vi "WhiteScreenTest_Startup.vi"() -> (0 "ErrorOut":errorcluster)   [LabVIEW 2018] (continued)
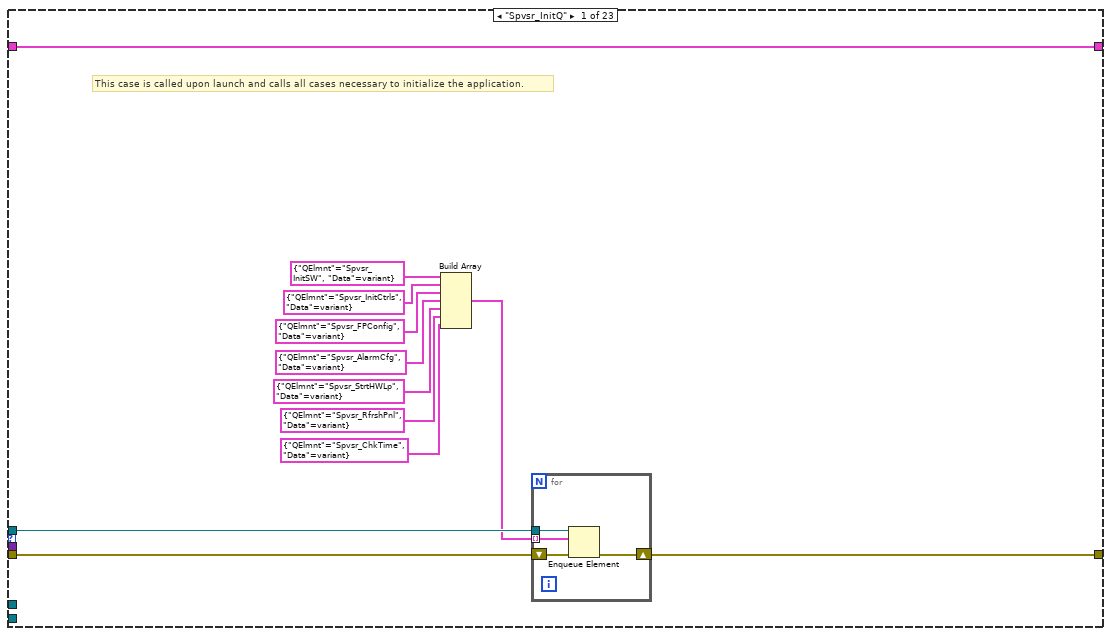
[diagram p6: hidden frame]
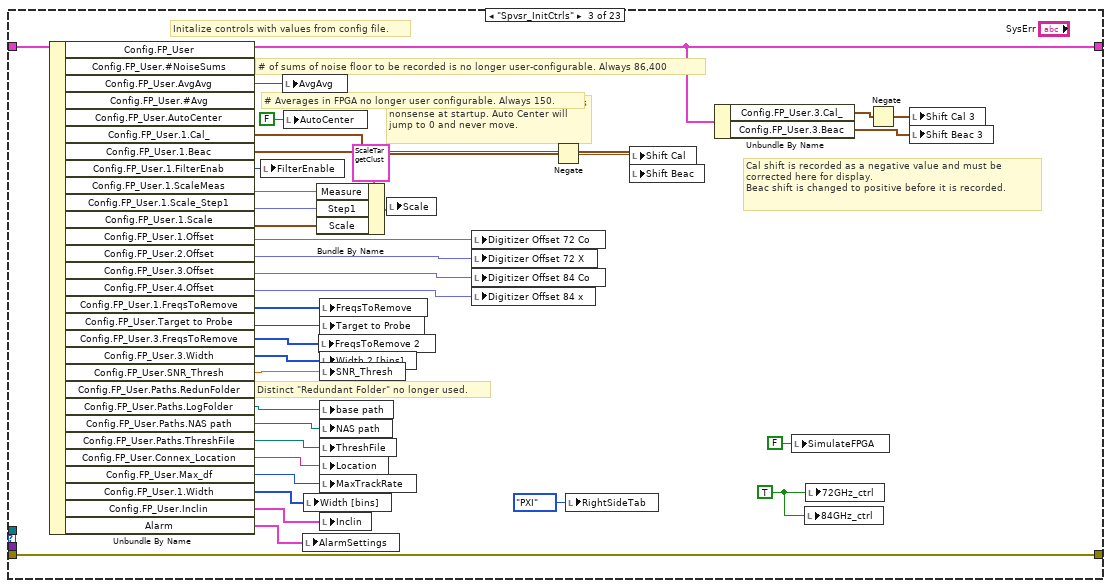
[diagram p9: hidden frame]
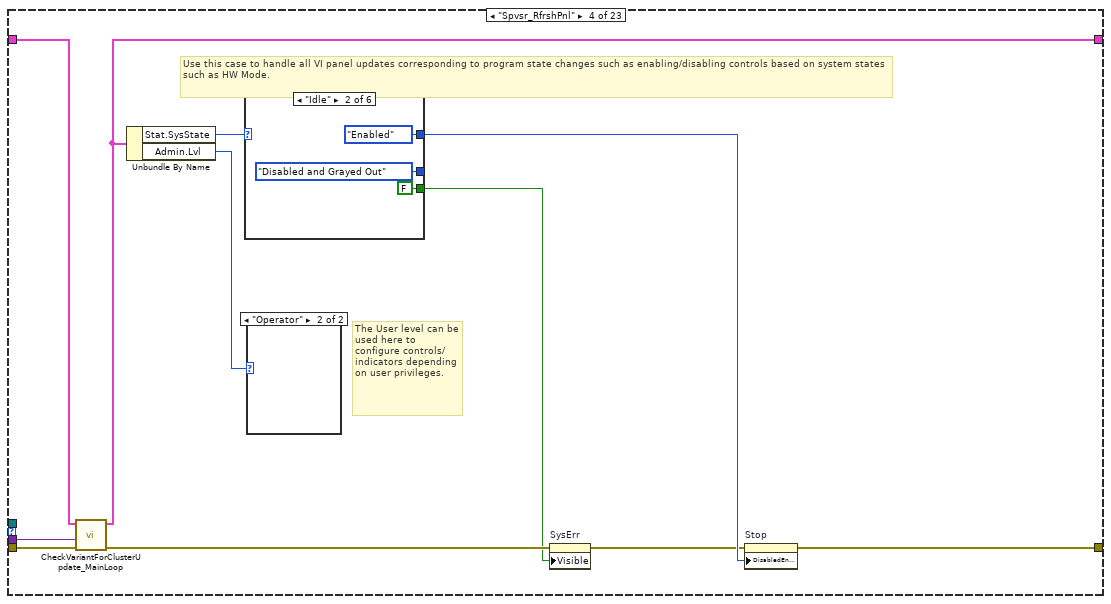
[diagram p10: hidden frame]
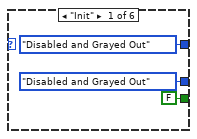
[diagram p12: hidden frame]
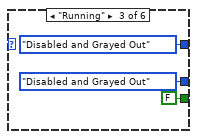
[diagram p13: hidden frame]
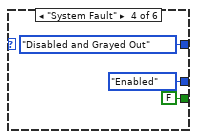
[diagram p14: hidden frame]
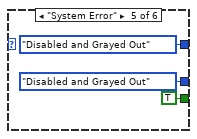
[diagram p15: hidden frame]
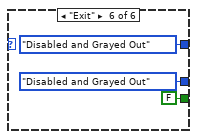
[diagram p16: hidden frame]
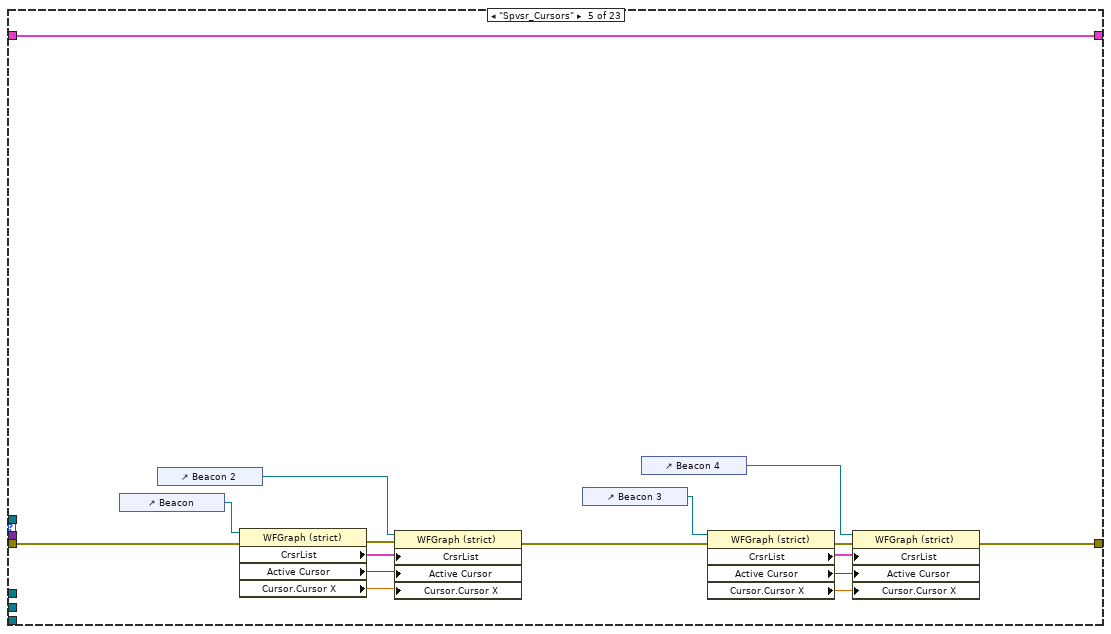
[diagram p17: hidden frame]
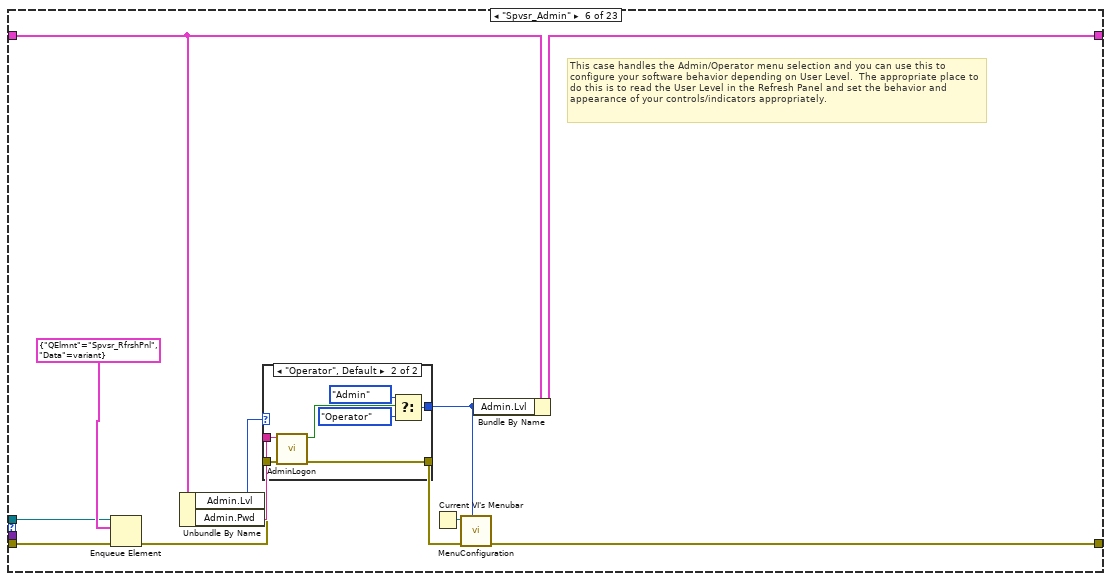
[diagram p18: hidden frame]
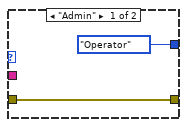
[diagram p19: hidden frame]
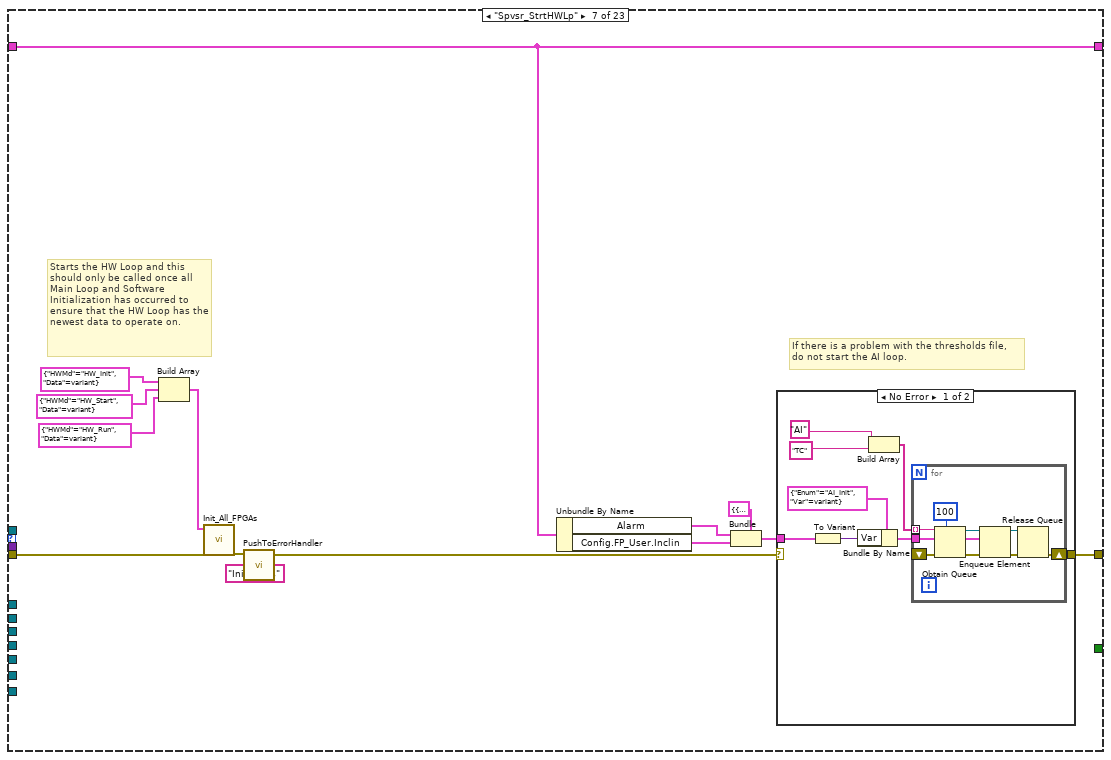
[diagram p20: hidden frame]
            n523 = Bundle By Name(cluster=w1148, "NoiseFloorSums.3"=w1146) -> (w1147:T24)
          }
          frame "4" {
            n524 = Unbundle By Name(w1155) -> ("AvgAvgSpectrum"=→"NoiseFloor 4":dbl[], "Sum"=w1151:dbl)  [unwired: 3 out]
            "NoiseFloorSum 4" <- w1151
            n525 = Bundle By Name(cluster=w1153, "NoiseFloorSums.4"=w1151) -> (w1152:T24)
          }
        }
      }
      frame "FP_Probes" {
        n526 = Variant To Data(error in=w1181, type=T60 {"Probe 1"=0, "Probe 2"=0.0, "Probe 3"=0.0, "Probe 4"=0.0, "Probe 5"=0.0, "Probe 6"=0.0, "Probe 7"=0.0, "Probe 7_1"=0.0, "IProbe"={"Probe 8"=0.0, "Probe 9"=0.0, "Probe 10"=0.0, "Probe 11"=0.0, "Probe 12"=0.0, "Probe 13"=0.0, "Probe 14"=0.0, "Probe 15"=0.0, "Probe 16"=0.0, "Probe 17"=0.0, "Probe 18"=0.0, "Probe 19"=0.0, "Probe20"=0.0}, "Probe 21"=0.0, "Probe 22"=0.0, "Probe 23"=0.0, "Probe 24"=0.0, "Probe Offsetd"=0.0, "CalShiftProbe"=0.0, "QProbe"={"Probe 8"=0.0, "Probe 9"=0.0, "Probe 10"=0.0, "Probe 11"=0.0, "Probe 12"=0.0, "Probe 13"=0.0, "Probe 14"=0.0, "Probe 15"=0.0, "Probe 16"=0.0, "Probe 17"=0.0, "Probe 18"=0.0, "Probe 19"=0.0, "Probe20"=0.0}, "AI_Over"=FALSE, "10MHzLocked"=FALSE} ("FPGA_Probes"), Variant=w1179) -> (data=w1178:T60, error out=w1182:errorcluster)
        n527 = Unbundle By Name(w1178) -> ("Probe 1"=→"Probe 1":i16, "Probe 2"=→"Probe 2":fxp<+/-,16,16>, "Probe 3"=→"Probe 3":fxp<+/-,39,24>, "Probe 5"=→"Probe 5":fxp<+/-,16,2>, "Probe 7"=→"Probe 7":fxp<+/-,18,1>, "IProbe"=→"I Probes":T20, "Probe 21"=→"Probe 21":fxp<+/-,24,5>, "Probe 22"=→"Probe 22":fxp<+/-,54,35>, "Probe 23"=→"Probe 23":fxp<+/-,54,1>, "Probe 24"=→"Probe 24":fxp<+/-,16,1>, "Probe Offsetd"=→"Probe Offsetd":fxp<+/-,16,16>, "QProbe"=→"Q Probes":T20, "AI_Over"=w1158:bool, "10MHzLocked"=→"10 MHzPLL Status":bool)
        n528 = First Call?() -> (First Call?: T/F=w1160:bool)
        n529 = Select(t=6.0 ("Set Start Time (s)"), s=w1160, f=0.0) -> (s? t:f=w1161:dbl)
        n530 = call "Elapsed Time6"("Time Target (s)"=5.0, "Reset"=w1158, "Set Start Time (s)"=w1161) -> ("Time has Elapsed"=w1159:bool)  [unwired: 9 in, 7 out]
        n531 = Not(x=w1159) -> (.not. x?=→"Input Over Range":bool)
      }
      frame "FP_PXI" {
        n532 = Variant To Data(error in=w1191, type=T61 {"Temperatures"=[], "Fans"=[], "Voltages"=[]} ("PXI"), Variant=w1189) -> (data=w1187:T61, error out=w1190:errorcluster)
        n533 = Unbundle By Name(w1187) -> ("Temperatures"=→"Temperatures":string[][], "Fans"=→"Fans":string[][], "Voltages"=→"Voltages":string[][])
      }
      frame "FP_AI" {
        w1201 = T65 {"RX?"=FALSE, "Warn"=FALSE, "Error"=FALSE, "Enabl"=FALSE, "Source"=""} ("element")
        # "Padding with \"no error\" because there are a few controls at the end that don't have error conditions."
        n534 = Variant To Data(error in=w1229, type=T62 {"AI"={"TimeString"="", "Time Stamp"=0.0, "AI0_Unused"=0.0, "AI1_-5V"=0.0, "AI2_+5V"=0.0, "AI3_+6V"=0.0, "AI4_+12V"=0.0, "AI5_+15V"=0.0, "AI6_+28V"=0.0, "AI7_Unused"=0.0, "Ai16_72GHz_CalPower"=0.0, "Ai17_84GHz_CalPower"=0.0, "Ai18_InclinAz"=0.0, "Ai19_InclinEl"=0.0, "Ai20_BlowerPwr"=0.0, "Ai21_Unused"=0.0, "Ai22_Unused"=0.0, "Ai23_Unused"=0.0, "InclinA_StdDev"=0.0, "InclinB_StdDev"=0.0, "InclinAz_Unfilt"=0.0, "InclinEl_Unfilt"=0.0}, "AllErrorStatus"={"AI 0"={"RX?"=FALSE, "Warn"=FALSE, "Error"=FALSE, "Enabl"=FALSE, "Source"=""}, "AI 1"={"RX?"=FALSE, "Warn"=FALSE, "Error"=FALSE, "Enabl"=FALSE, "Source"=""}, "AI 2"={"RX?"=FALSE, "Warn"=FALSE, "Error"=FALSE, "Enabl"=FALSE, "Source"=""}, "AI 3"={"RX?"=FALSE, "Warn"=FALSE, "Error"=FALSE, "Enabl"=FALSE, "Source"=""}, "AI 4"={"RX?"=FALSE, "Warn"=FALSE, "Error"=FALSE, "Enabl"=FALSE, "Source"=""}, "AI 5"={"RX?"=FALSE, "Warn"=FALSE, "Error"=FALSE, "Enabl"=FALSE, "Source"=""}, "AI 6"={"RX?"=FALSE, "Warn"=FALSE, "Error"=FALSE, "Enabl"=FALSE, "Source"=""}, "AI 7"={"RX?"=FALSE, "Warn"=FALSE, "Error"=FALSE, "Enabl"=FALSE, "Source"=""}, "AI 16"={"RX?"=FALSE, "Warn"=FALSE, "Error"=FALSE, "Enabl"=FALSE, "Source"=""}, "AI 17"={"RX?"=FALSE, "Warn"=FALSE, "Error"=FALSE, "Enabl"=FALSE, "Source"=""}, "AI 18"={"RX?"=FALSE, "Warn"=FALSE, "Error"=FALSE, "Enabl"=FALSE, "Source"=""}, "AI 19"={"RX?"=FALSE, "Warn"=FALSE, "Error"=FALSE, "Enabl"=FALSE, "Source"=""}, "AI 20"={"RX?"=FALSE, "Warn"=FALSE, "Error"=FALSE, "Enabl"=FALSE, "Source"=""}, "AI 21"={"RX?"=FALSE, "Warn"=FALSE, "Error"=FALSE, "Enabl"=FALSE, "Source"=""}, "AI 22"={"RX?"=FALSE, "Warn"=FALSE, "Error"=FALSE, "Enabl"=FALSE, "Source"=""}, "AI 23"={"RX?"=FALSE, "Warn"=FALSE, "Error"=FALSE, "Enabl"=FALSE, "Source"=""}}}, Variant=w1227) -> (data=w1225:T62, error out=w1228:errorcluster)
        n535 = Unbundle By Name(w1225) -> ("AI"=w1222:T63, "AllErrorStatus"=w1223:T64)
        n536 = Unbundle By Name(w1223) -> ("AI 0"=w1221:T65, "AI 1"=w1219:T65, "AI 2"=w1218:T65, "AI 3"=w1217:T65, "AI 4"=w1216:T65, "AI 5"=w1215:T65, "AI 6"=w1214:T65, "AI 16"=w1213:T65, "AI 17"=w1212:T65, "AI 18"=w1211:T65, "AI 19"=w1210:T65)  [unwired: 1 out]
        n537 = call "SortVoltage_Display.vi"("Voltage"=w1222) -> ("VoltageDisplay"=w1200:T15)  [unwired: 10 in]
        "VoltageDisplay" <- w1200
        n538 = Build Array(w1221, w1219, w1218, w1217, w1216, w1215, w1214, w1213, w1212, w1211, w1210, w1201, w1201, w1201, w1201) -> (w1220:T65[])
        n539 = control-ref of="VoltageDisplay"() -> (w1209:refnum<vi>)
        n540 = property on="Property Node" class="Clust (strict)"(reference=w1209) -> ("Controls[]"=w1224:refnum<vi>[])  [unwired: 1 in, 2 out]
        n541 = Unbundle By Name(w1200) -> ("Ai18_InclinometerAz"=w1208:dbl, "Ai19_InclinometerEl"=w1207:dbl)
        n542 = for {
          tunnel: w1224 -> [w1234] mode=indexing
          tunnel: w1220 -> [w1231] mode=indexing
          n543 = call "Indicator_Error_Color.vi"("AI 0"=w1231) -> ("Label.Text Colors:BG Color"=w1230:u32)  [unwired: 10 in]
          n544 = To More Specific Class(target class=refnum<vi> refnum ("AI0_Inclinometer"), reference=w1234) -> (specific class reference=w1233:refnum<vi>)  [unwired: 1 in, 1 out]
          n545 = property on="Property Node" class="DigNum"(reference=w1233, "NumText.BGColor"=w1230) -> ()  [unwired: 1 in, 2 out]
        }
        n546 = Unbundle By Name(w1200) -> ("Az_StdDev"=w1205:dbl, "El_StdDev"=w1204:dbl)
        n547 = Bundle("Ai18_InclinometerAz"=w1208, "Ai19_InclinometerEl"=w1207) -> (→"Inclinometer History":T14)  [unwired: 1 in]
        n548 = Bundle("Az_StdDev"=w1205, "El_StdDev"=w1204) -> (→"Inclinometer Std Dev History":cluster{"Az_StdDev":dbl, "El_StdDev":dbl})  [unwired: 1 in]
        n549 = Unbundle By Name(w1200) -> ("AI1_-5V"=→"-5V":dbl, "AI2_+5V"=→"+5":dbl, "AI3_+6V"=→"+6":dbl, "AI4_+12V"=→"+12":dbl, "AI5_+15V"=→"+15":dbl, "AI6_+28V"=→"+28":dbl, "Ai18_InclinometerAz"=→"InclAz":dbl, "Ai19_InclinometerEl"=→"InclEl":dbl)  [unwired: 2 out]
      }
      frame "FP_TC" {
        n550 = Variant To Data(error in=w1264, type=T66 {"TCData"={"TimeStamp"=0.0, "TimeString"="", "TC0_LP1_Hi"=0.0, "TC1_LP1_MidHi"=0.0, "TC2_LP1_Mid"=0.0, "TC3_LP1_LoMid"=0.0, "TC4_LP1_Lo"=0.0, "TC5_LP2_Hi"=0.0, "TC6_LP2_MidHi"=0.0, "TC7_LP2_Mid"=0.0, "TC8_LP2_LoMid"=0.0, "TC9_LP2_Lo"=0.0, "TC10_HVAC_Cond_In"=0.0, "TC11_HVAC_Cond_Out"=0.0, "TC12_Gen_Exhaust"=0.0, "TC13_Unused"=0.0, "TC14_Unused"=0.0, "TC15_Unused"=0.0, "TC16_Unused"=0.0, "TC17_Unused"=0.0, "TC18_Unused"=0.0, "TC19_Unused"=0.0, "TC20_Unused"=0.0, "TC21_Unused"=0.0, "TC22_Unused"=0.0, "TC23_Unused"=0.0, "TC24_Unused"=0.0, "TC25_Unused"=0.0, "TC26_Unused"=0.0, "TC27_Unused"=0.0, "TC28_Unused"=0.0, "TC29_Unused"=0.0, "TC30_Unused"=0.0, "TC31_Unused"=0.0}, "All_TC_ErrorStatus"={"TC 0"={"RX?"=FALSE, "Warn"=FALSE, "Error"=FALSE, "Enabl"=FALSE, "Source"=""}, "TC 1"={"RX?"=FALSE, "Warn"=FALSE, "Error"=FALSE, "Enabl"=FALSE, "Source"=""}, "TC 2"={"RX?"=FALSE, "Warn"=FALSE, "Error"=FALSE, "Enabl"=FALSE, "Source"=""}, "TC 3"={"RX?"=FALSE, "Warn"=FALSE, "Error"=FALSE, "Enabl"=FALSE, "Source"=""}, "TC 4"={"RX?"=FALSE, "Warn"=FALSE, "Error"=FALSE, "Enabl"=FALSE, "Source"=""}, "TC 5"={"RX?"=FALSE, "Warn"=FALSE, "Error"=FALSE, "Enabl"=FALSE, "Source"=""}, "TC 6"={"RX?"=FALSE, "Warn"=FALSE, "Error"=FALSE, "Enabl"=FALSE, "Source"=""}, "TC 7"={"RX?"=FALSE, "Warn"=FALSE, "Error"=FALSE, "Enabl"=FALSE, "Source"=""}, "TC 8"={"RX?"=FALSE, "Warn"=FALSE, "Error"=FALSE, "Enabl"=FALSE, "Source"=""}, "TC 9"={"RX?"=FALSE, "Warn"=FALSE, "Error"=FALSE, "Enabl"=FALSE, "Source"=""}, "TC 10"={"RX?"=FALSE, "Warn"=FALSE, "Error"=FALSE, "Enabl"=FALSE, "Source"=""}, "TC 11"={"RX?"=FALSE, "Warn"=FALSE, "Error"=FALSE, "Enabl"=FALSE, "Source"=""}, "TC 12"={"RX?"=FALSE, "Warn"=FALSE, "Error"=FALSE, "Enabl"=FALSE, "Source"=""}, "TC 13"={"RX?"=FALSE, "Warn"=FALSE, "Error"=FALSE, "Enabl"=FALSE, "Source"=""}, "TC 14"={"RX?"=FALSE, "Warn"=FALSE, "Error"=FALSE, "Enabl"=FALSE, "Source"=""}, "TC 15"={"RX?"=FALSE, "Warn"=FALSE, "Error"=FALSE, "Enabl"=FALSE, "Source"=""}, "TC 16"={"RX?"=FALSE, "Warn"=FALSE, "Error"=FALSE, "Enabl"=FALSE, "Source"=""}, "TC 17"={"RX?"=FALSE, "Warn"=FALSE, "Error"=FALSE, "Enabl"=FALSE, "Source"=""}, "TC 18"={"RX?"=FALSE, "Warn"=FALSE, "Error"=FALSE, "Enabl"=FALSE, "Source"=""}, "TC 19"={"RX?"=FALSE, "Warn"=FALSE, "Error"=FALSE, "Enabl"=FALSE, "Source"=""}, "TC 20"={"RX?"=FALSE, "Warn"=FALSE, "Error"=FALSE, "Enabl"=FALSE, "Source"=""}}}, Variant=w1263) -> (data=w1261:T66, error out=w1237:errorcluster)
        n551 = Unbundle By Name(w1261) -> ("TCData"=w1260:T67, "All_TC_ErrorStatus"=w1243:T68)
        n552 = Unbundle By Name(w1243) -> ("TC 0"=w1254:T65, "TC 1"=w1253:T65, "TC 2"=w1252:T65, "TC 3"=w1251:T65, "TC 4"=w1250:T65, "TC 5"=w1249:T65, "TC 6"=w1248:T65, "TC 7"=w1241:T65, "TC 8"=w1247:T65, "TC 9"=w1246:T65, "TC 10"=w1245:T65, "TC 11"=w1244:T65, "TC 12"=w1240:T65, "TC 13"=w1239:T65)
        n553 = call "SortTC_Display.vi"("TCData"=w1260) -> ("TCsDisplay"=w1236:T16)  [unwired: 10 in]
        "TCsDisplay" <- w1236
        n554 = control-ref of="TCsDisplay"() -> (w1238:refnum<vi>)
        n555 = property on="Property Node" class="Clust (strict)"(reference=w1238) -> ("Controls[]"=w1259:refnum<vi>[])  [unwired: 1 in, 2 out]
        n556 = Build Array(w1254, w1253, w1252, w1251, w1250, w1249, w1248, w1241, w1247, w1246, w1245, w1244, w1240, w1239) -> (w1242:T65[])
        n557 = Unbundle By Name(w1236) -> ("TC13_Tamb_Interior"=→"ConnextIntTemp":dbl)
        n558 = Delete From Array(array=w1259, length=2, index=0) -> (array with subset deleted=w1258:refnum<vi>[])  [unwired: 1 out]
        n559 = for {
          tunnel: w1258 -> [w1269] mode=indexing
          tunnel: w1242 -> [w1265] mode=indexing
          n560 = To More Specific Class(target class=refnum<vi> refnum ("AI0_Inclinometer"), reference=w1269) -> (specific class reference=w1268:refnum<vi>)  [unwired: 1 in, 1 out]
          n561 = call "Indicator_Error_Color.vi"("AI 0"=w1265) -> ("Label.Text Colors:BG Color"=w1266:u32)  [unwired: 10 in]
          n562 = property on="Property Node" class="DigNum"(reference=w1268, "NumText.BGColor"=w1266) -> ()  [unwired: 1 in, 2 out]
        }
      }
      frame "FP_PWR_Hist" {
        n563 = Unbundle By Name(w1283) -> ("PwrHist.72Co"=w1282:T13, "PwrHist.72X"=w1281:T13, "PwrHist.84Co"=w1280:T13, "PwrHist.84X"=w1279:T13)
        n564 = Unbundle By Name(w1282) -> ("Cal Smooth"=w1278:dbl, "Beac Smooth"=w1277:dbl)
        n565 = Unbundle By Name(w1281) -> ("Cal Smooth"=w1276:dbl, "Beac Smooth"=w1275:dbl)
        n566 = Unbundle By Name(w1280) -> ("Cal Smooth"=w1274:dbl, "Beac Smooth"=w1273:dbl)
        n567 = Unbundle By Name(w1279) -> ("Cal Smooth"=w1272:dbl, "Beac Smooth"=w1271:dbl)
        n568 = Bundle("Cal Smooth"=w1278, "Beac Smooth"=w1277, "Cal Smooth"=w1276, "Beac Smooth"=w1275, "Cal Smooth"=w1274, "Beac Smooth"=w1273, "Cal Smooth"=w1272, "Beac Smooth"=w1271) -> (→"Combined Power History":T7)  [unwired: 1 in]
      }
      frame "FP_Alarm" {
        w1312 = refnum<vi> refnum ("element")
        # "0: TC13\n1-8: AI1-6,18-19\n9-11: TE1-TE3\n12-15: ADAM1-ADAM4\n\n16: 72Co BeacFreq\n17: Placeholder\n18: 84 Co BeacFreq\n19: Placeholder\n \n20: 72Co CalFreq\n21: Placeholder\n22: 84Co CalFreq\n23: Placeholder\n \n24: 72Co CalTonePwr\n25: 72X CalTonePwr\n26: 84Co CalTonePwr\n27: 84X CalTonePwr\n\n28: SNR Timer"
        # "From Log Loop"
        n569 = Variant To Data(error in=w1351, type=T69 {"Alarms"={"Green"=TRUE, "Rx_Yell"=FALSE, "Cx_Yell"=FALSE, "Red"=FALSE, "Source"=""}, "SerialMeas"={"TE_Air"=0.0, "TE_Bottom"=0.0, "TE_Front"=0.0, "ADAM-Co"=0.0, "ADAM-XPol"=0.0, "ADAM-CalEncl"=0.0, "ADAM-Noise"=0.0}, "AllAlarms"=[], "Elapsed_SNR_Timer"=0.0, "Saturation"={"84"=[], "72"=[]}}, Variant=w1350) -> (data=w1349:T69, error out=w1299:errorcluster)
        n570 = Unbundle By Name(w1349) -> ("Elapsed_SNR_Timer"=→"Elapsed_SNR_Timer":dbl, "Alarms"=→"Alarms":T1, "AllAlarms"=w1339:T65[], "SerialMeas"=w1348:T70, "Saturation"=w1285:T71)
        n571 = control-ref of="MeasMax"() -> (w1306:refnum<vi>)
        n572 = control-ref of="1_Max"() -> (w1305:refnum<vi>)
        n573 = control-ref of="4_Max"() -> (w1304:refnum<vi>)
        n574 = control-ref of="5_Max"() -> (w1303:refnum<vi>)
        n575 = control-ref of="6_Max"() -> (w1302:refnum<vi>)
        n576 = control-ref of="7_Max"() -> (w1301:refnum<vi>)
        n577 = Unbundle By Name(w1348) -> ("TE_Air"=→"TE_Air":dbl, "TE_Bottom"=→"TE_Bottom":dbl, "TE_Front"=→"TE_Front":dbl, "ADAM-Co"=→"ADAM-Co":dbl, "ADAM-XPol"=→"ADAM-XPol":dbl, "ADAM-CalEncl"=→"ADAM-CalEncl":dbl, "ADAM-Noise"=→"ADAM-Noise":dbl)
        n578 = Unbundle By Name(w1285) -> ("84"=w1297:bool[])
        n579 = Build Array(w1306, w1305, w1304, w1303, w1302, w1301) -> (w1300:refnum<vi>[])
        n580 = call "Saturation_Indicator_Color_Code.vi"("SaturationStatus"=w1297, "IndicatorRefs"=w1300) -> ("Error"=w1288:errorcluster)  [unwired: 9 in]
        n581 = control-ref of="MeasMax"() -> (w1289:refnum<vi>)
        n582 = control-ref of="1_Max"() -> (w1290:refnum<vi>)
        n583 = control-ref of="4_Max"() -> (w1291:refnum<vi>)
        n584 = control-ref of="5_Max"() -> (w1292:refnum<vi>)
        n585 = control-ref of="6_Max"() -> (w1293:refnum<vi>)
        n586 = control-ref of="7_Max"() -> (w1294:refnum<vi>)
        n587 = Unbundle By Name(w1285) -> ("72"=w1296:bool[])
        n588 = Build Array(w1289, w1290, w1291, w1292, w1293, w1294) -> (w1295:refnum<vi>[])
        n589 = control-ref of="ConnextIntTemp"() -> (w1328:refnum<vi>)
        n590 = control-ref of="-5V"() -> (w1329:refnum<vi>)
        n591 = control-ref of="+5"() -> (w1330:refnum<vi>)
        n592 = control-ref of="+6"() -> (w1331:refnum<vi>)
        n593 = control-ref of="+12"() -> (w1332:refnum<vi>)
        n594 = control-ref of="+15"() -> (w1333:refnum<vi>)
        n595 = control-ref of="+28"() -> (w1334:refnum<vi>)
        n596 = control-ref of="InclAz"() -> (w1335:refnum<vi>)
        n597 = control-ref of="InclEl"() -> (w1336:refnum<vi>)
        n598 = control-ref of="TE_Air"() -> (w1337:refnum<vi>)
        n599 = control-ref of="TE_Bottom"() -> (w1326:refnum<vi>)
        n600 = control-ref of="TE_Front"() -> (w1319:refnum<vi>)
        n601 = call "Saturation_Indicator_Color_Code.vi"("SaturationStatus"=w1296, "IndicatorRefs"=w1295) -> ("Error"=w1287:errorcluster)  [unwired: 9 in]
        n602 = Merge Errors(w1288, w1287) -> (w1286:errorcluster)
        n603 = Build Array(w1328, w1329, w1330, w1331, w1332, w1333, w1334, w1335, w1336, w1337, w1326, w1319) -> (w1322:refnum<vi>[])
        n604 = control-ref of="ADAM-Co"() -> (w1327:refnum<vi>)
        n605 = control-ref of="ADAM-XPol"() -> (w1325:refnum<vi>)
        n606 = control-ref of="ADAM-CalEncl"() -> (w1324:refnum<vi>)
        n607 = control-ref of="ADAM-Noise"() -> (w1323:refnum<vi>)
        n608 = control-ref of="72CoBeacFrq"() -> (w1318:refnum<vi>)
        n609 = control-ref of="84CoBeacFrq"() -> (w1315:refnum<vi>)
        n610 = control-ref of="72CoCalFrq"() -> (w1314:refnum<vi>)
        n611 = control-ref of="84CoCalFrq"() -> (w1313:refnum<vi>)
        n612 = control-ref of="MaxValue_Cal_72Co"() -> (w1311:refnum<vi>)
        n613 = control-ref of="MaxValue_Cal_72X"() -> (w1310:refnum<vi>)
        n614 = control-ref of="MaxValue_Cal_84Co"() -> (w1309:refnum<vi>)
        n615 = control-ref of="MaxValue_Cal_84X"() -> (w1308:refnum<vi>)
        n616 = control-ref of="Elapsed_SNR_Timer"() -> (w1316:refnum<vi>)
        n617 = Build Array(w1327, w1325, w1324, w1323, w1318, w1312, w1315, w1312, w1314, w1312, w1313, w1312, w1311, w1310, w1309, w1308, w1316) -> (w1321:refnum<vi>[])
        n618 = Build Array (concatenate)(w1322, w1321) -> (w1320:refnum<vi>[])
        n619 = Merge Errors(w1286, w1299) -> (w1298:errorcluster)
        n620 = for {
          tunnel: w1320 -> [w1361] mode=indexing
          tunnel: w1339 -> [w1357] mode=indexing
          shift-right: [w1354] -> w1338
          shift-left: w1298 -> [w1353]
          n621 = To More Specific Class(target class=refnum<vi> refnum ("AI0_Inclinometer"), reference=w1361) -> (specific class reference=w1360:refnum<vi>, error out=w1355:errorcluster)  [unwired: 1 in]
          n622 = call "Indicator_Error_Color.vi"("AI 0"=w1357) -> ("Label.Text Colors:BG Color"=w1358:u32)  [unwired: 10 in]
          n623 = property on="Property Node" class="DigNum"(reference=w1360, error in=w1355, "NumText.BGColor"=w1358) -> (error out=w1356:errorcluster)  [unwired: 1 out]
          n624 = Merge Errors(w1353, w1356) -> (w1354:errorcluster)
        }
      }
      frame "FP_Exit" {
        n625 = Release Queue(queue=w1365, error in (no error)=w1364) -> (error out=w1363:errorcluster)  [unwired: 1 in, 2 out]
      }
    }
    "FP_Count" <- w912
  }
  n626 = disable-structure shown="Enabled" {
    disable-tunnel: w131 -> [w1372 w1373]
    disable-tunnel: w53 -> [w1371 _]
    disable-tunnel: [w1370 w1373] -> w123
    disable-tunnel: w114 -> [w1369 _]
    disable-tunnel: TargetNumber."2" ("FPGA.Target") -> [w1368 _]
    disable-tunnel: w64 -> [w1367 _]
    frame Enabled {
      n627 = call "HW_Loop_20181101.vi"("ErrorLocation"=w1369, "error in (no error)"=w1372, "10MHzPLL?"=w1367, "FPGA.Target"=w1368, "Queue in"=w1371) -> ("error out"=w1370:errorcluster)  [unwired: 6 in]
    }
    frame Disabled {
    }
  }
  n628 = call "HW_Loop_20181101.vi"("ErrorLocation"=w115, "error in (no error)"=w149, "10MHzPLL?"=w64, "FPGA.Target"=TargetNumber."1", "Queue in"=w150) -> ("error out"=w148:errorcluster)  [unwired: 6 in]
  n629 = property class="VI"(error in=w41) -> (error out=w48:errorcluster, "Panel"=w46:refnum<vi>)  [unwired: 1 in, 1 out]
  n630 = disable-structure shown="Enabled" {
    disable-tunnel: [w1375 w1376] -> w113
    disable-tunnel: w57 -> [w1374 w1376]
    frame Enabled {
      n631 = call "PXI_Health_Loop.vi"("error in (no error)"=w1374) -> ("error out"=w1375:errorcluster)  [unwired: 10 in]
    }
    frame Disabled {
    }
  }
  n632 = property class="VI"(error in=w5) -> (error out=w13:errorcluster, "Panel"=w15:refnum<vi>)  [unwired: 1 in, 1 out]
  n633 = property class="VI"(error in=w31) -> (error out=w38:errorcluster, "Panel"=w40:refnum<vi>)  [unwired: 1 in, 1 out]
  n634 = property class="VI"(error in=w17) -> (error out=w25:errorcluster, "Panel"=w27:refnum<vi>)  [unwired: 1 in, 1 out]
  n635 = property class="Pnl"(reference=w46, error in=w48) -> (reference out=w47:refnum<vi>, error out=w49:errorcluster, "Panes[]"=w52:refnum<vi>[])
  n636 = property class="Pnl"(reference=w15, error in=w13) -> (reference out=w14:refnum<vi>, error out=w12:errorcluster, "Panes[]"=w9:refnum<vi>[])
  n637 = property class="Pnl"(reference=w40, error in=w38) -> (reference out=w39:refnum<vi>, error out=w37:errorcluster, "Panes[]"=w34:refnum<vi>[])
  n638 = property class="Pnl"(reference=w27, error in=w25) -> (reference out=w26:refnum<vi>, error out=w24:errorcluster, "Panes[]"=w21:refnum<vi>[])
  n639 = Close Reference(reference=w47, error in (no error)=w49) -> (error out=w50:errorcluster)
  n640 = Close Reference(reference=w14, error in (no error)=w12) -> (error out=w11:errorcluster)
  n641 = Close Reference(reference=w39, error in (no error)=w37) -> (error out=w36:errorcluster)
  n642 = Close Reference(reference=w26, error in (no error)=w24) -> (error out=w23:errorcluster)
  n643 = for {
    tunnel: w52 -> [w1380] mode=indexing
    tunnel: w50 -> [w1379]
    shift-right: [w1378] -> w51
    shift-left: _ -> [_]
    w1377 = T73."Off While Running" ("Horizontal Scrollbar Visibility")
    n644 = property class="Pane"(reference=w1380, error in=w1379, "HorizScrollbarVisibility"=w1377, "VertScrollbarVisibility"=w1377) -> (error out=w1378:errorcluster)  [unwired: 1 out]
  }
  n645 = for {
    tunnel: w9 -> [w1384] mode=indexing
    tunnel: w11 -> [w1383]
    shift-right: [w1382] -> w10
    shift-left: _ -> [_]
    w1381 = T73."Off While Running" ("Horizontal Scrollbar Visibility")
    n646 = property class="Pane"(reference=w1384, error in=w1383, "HorizScrollbarVisibility"=w1381, "VertScrollbarVisibility"=w1381) -> (error out=w1382:errorcluster)  [unwired: 1 out]
  }
  n647 = for {
    tunnel: w34 -> [w1388] mode=indexing
    tunnel: w36 -> [w1387]
    shift-right: [w1386] -> w35
    shift-left: _ -> [_]
    w1385 = T73."Off While Running" ("Horizontal Scrollbar Visibility")
    n648 = property class="Pane"(reference=w1388, error in=w1387, "HorizScrollbarVisibility"=w1385, "VertScrollbarVisibility"=w1385) -> (error out=w1386:errorcluster)  [unwired: 1 out]
  }
  n649 = for {
    tunnel: w21 -> [w1392] mode=indexing
    tunnel: w23 -> [w1391]
    shift-right: [w1390] -> w22
    shift-left: _ -> [_]
    w1389 = T73."Off While Running" ("Horizontal Scrollbar Visibility")
    n650 = property class="Pane"(reference=w1392, error in=w1391, "HorizScrollbarVisibility"=w1389, "VertScrollbarVisibility"=w1389) -> (error out=w1390:errorcluster)  [unwired: 1 out]
  }
  n651 = Close Reference(reference=w52, error in (no error)=w51) -> (error out=w105:errorcluster)
  n652 = Close Reference(reference=w9, error in (no error)=w10) -> (error out=w101:errorcluster)
  n653 = Close Reference(reference=w34, error in (no error)=w35) -> (error out=w109:errorcluster)
  n654 = Close Reference(reference=w21, error in (no error)=w22) -> (error out=w103:errorcluster)
  n655 = Build Array(w63, w62, w61) -> (w58:refnum<vi>[])
  n656 = Merge Errors(w155, w154, w148, w123, w146, w133, w143, w116, w107, w54, w117, w110, w113, w108, w109, w105, w103, w101, w104) -> (w60:errorcluster)
  n657 = call "Abort_NASA_VIs.vi"("error in"=w60, "VI_Refs"=w58) -> ("error out"=w59:errorcluster)  [unwired: 9 in]
  n658 = flat-sequence {
    tunnel: [w1393] -> w140
    tunnel: w59 -> [w1393]
    frame #0 {
      n659 = local write "Exit"(FALSE ("Exit")) -> ()
    }
  }
  n660 = disable-structure shown="Disabled" {
    frame Disabled {
    }
    frame Enabled {
    }
  }
  n661 = call "ExitLabVIEW.vi"("ErrorIn"=w140) -> ("ErrorOut"=→"ErrorOut":errorcluster)  [unwired: 14 out]
